vi "AlGaInPAs_prep_run_cont_dil_v13.vi"(2 "Debug Mode":bool, 3 "Elapsed Time(s)":dbl, 4 "State":enum16{"Edit", "Start", "Run", "End", "Idle"}(ring), 5 "Argument List In":string[](array[string])) -> (0 "Status Out":string, 1 "Argument List Out":string[](array[string]))   [LabVIEW 2011]
panel:
  out "Prep-In var":bool
  out "Prep-Ga var":bool
  out "Prep-Al var":bool
  out "Prep-P var":bool
  out "Prep-As var":bool
  out "prep_done":bool
  out "run started":bool
  out "first":bool=TRUE
  out "total time":dbl
  out "is OK?":bool
  out "AsH3?":bool
  out "PH3?":bool
  out "In?":bool
  out "Ga?":bool
  out "Al?":bool
  in  "Prep As":bool caption="Pre-run"
  in  "Prep P":bool caption="Pre-run"
  in  "Prep In":bool caption="Pre-run"
  in  "prep_time":dbl caption="pre-run time (s)"
  in  "Prep Al":bool caption="Pre-run"
  in  "Run As":bool caption="Run"
  in  "AsH3 Flow":dbl caption="AsH3 Flow (0-10 sccm)" format="%.2f"
  in  "P Flow":dbl caption="P Flow (0-100 sccm)" format="%.2f"
  in  "Run P":bool caption="Run"
  in  "In Flow":dbl caption="In Flow (0-100 sscm)" format="%.2f"
  in  "Run In":bool caption="Run"
  in  "Run Al":bool caption="Run"
  in  "Al Flow":dbl caption="Al Flow (0-100 sscm)" format="%.2f"
  in  "Cancel":bool
  in  "OK":bool
  out "tTotal(s) 2":dbl
  in  "Ga Tab Control":enum32{"Page 1", "Page 2", "Page 3"}(tab)
  in  "Ga Dilution":bool caption="Dilute"
  in  "Ga Flow set":dbl caption="Ga Flow (0-10 sscm)" format="%.2f"
  in  "Run Ga":bool caption="Run"
  in  "Prep Ga":bool caption="Pre-run"
  out "Ga Flow val":dbl caption="Ga Flow (0-10 sscm)" format="%.2f"
  in  "GAMFC1 set":dbl=1.0 caption="R1 (0-10 sscm)" format="%.2f"
  out "GAMFC2 val":dbl caption="R2 (0-100 sscm)" format="%.2f"
  in  "GAMFC3 set":dbl=100.0 caption="R3 (0-1000 sscm)" format="%.1f"
  out "GAMFC1 val":dbl caption="R1 (0-10 sscm)" format="%.2f"
  in  "GAMFC2 set":dbl caption="R2 (0-100 sscm)" format="%.2f"
  out "GAMFC3 val":dbl=100.0 caption="R3 (0-1000 sscm)" format="%.1f"
  in  "Ga calculated":u16(ring) items=["Ga flow", "MFC1", "MFC2", "MFC3"]
  # "Add pre-run time to run time in editor."
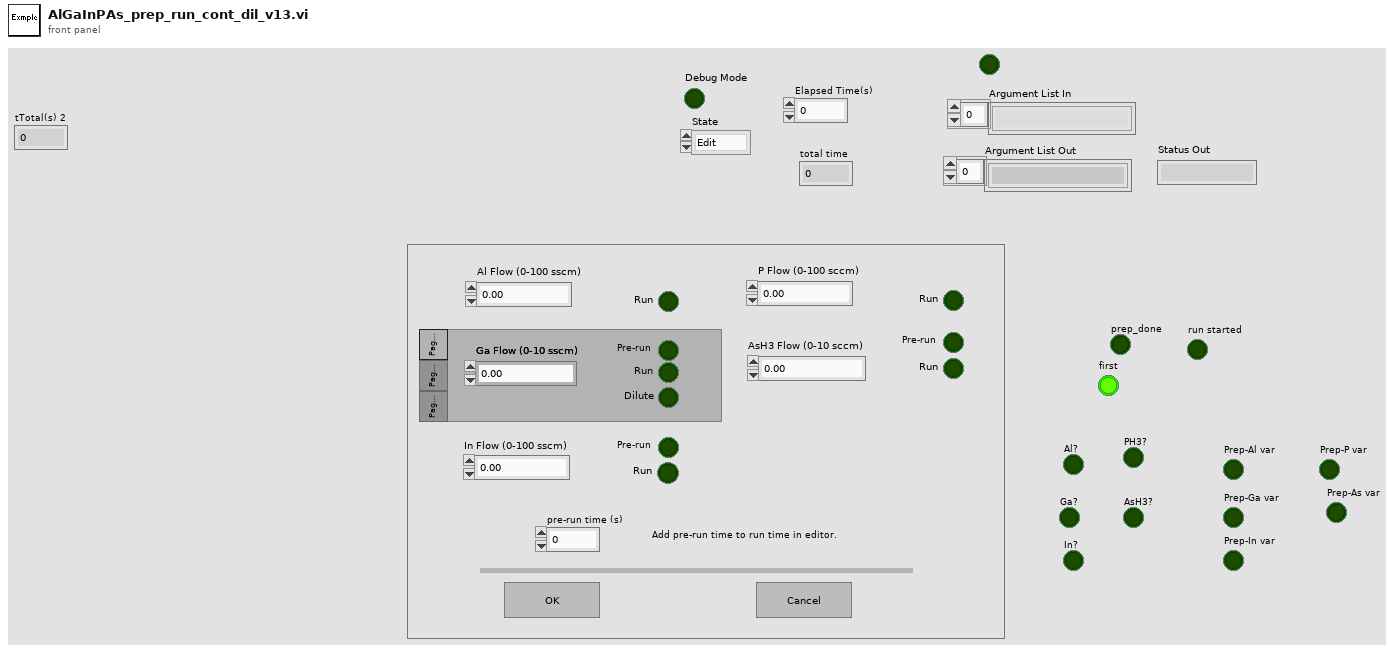
[diagram p1: front panel]
types:
  T1 = enum16{"Discrete", "Continuous", "Instantaneous", "Finite"}
  T2 = enum32{"Invalid", "Default", "Floating", "Floating/Auto-Hide", "Modal"}
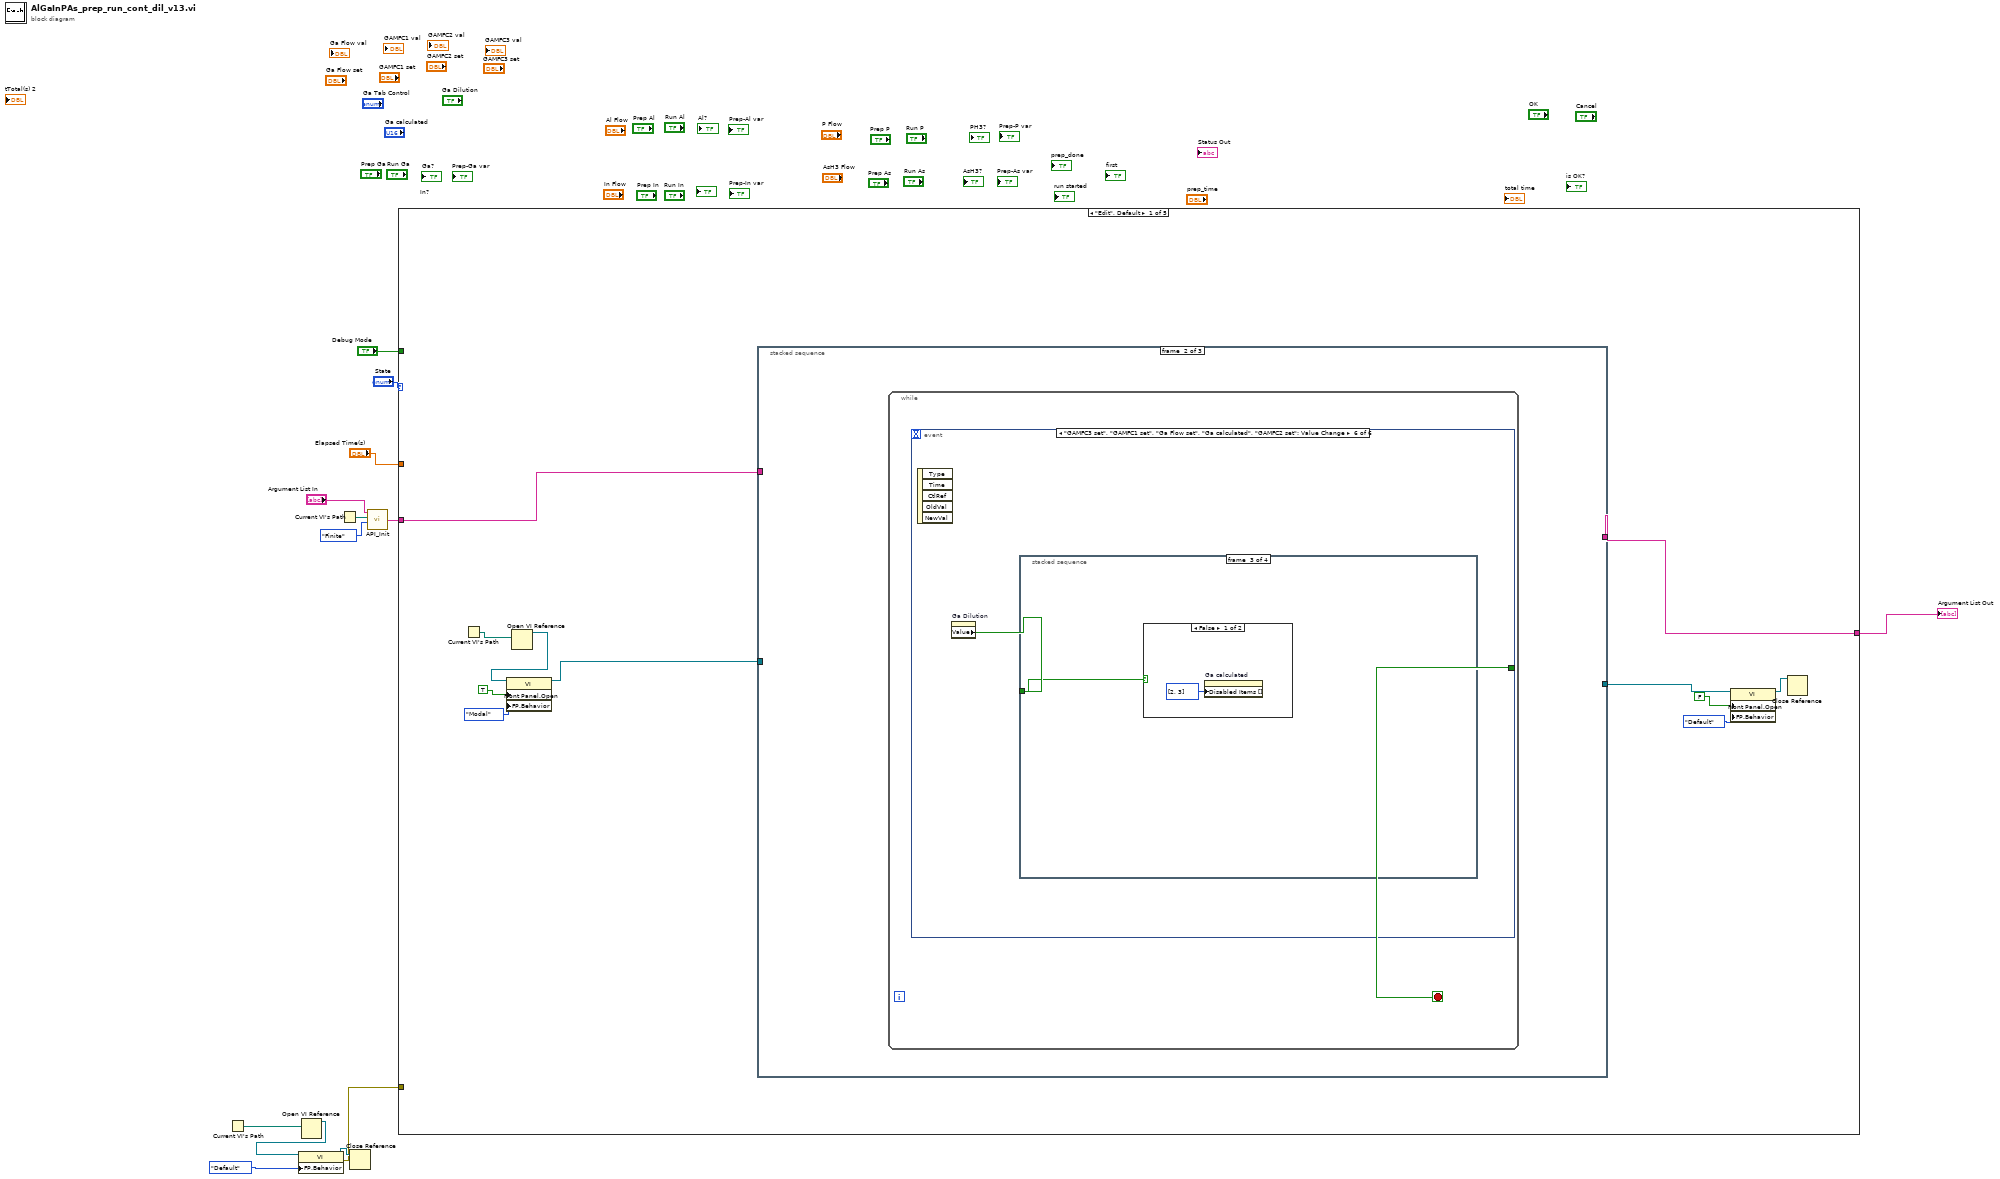
[diagram p0: block diagram]
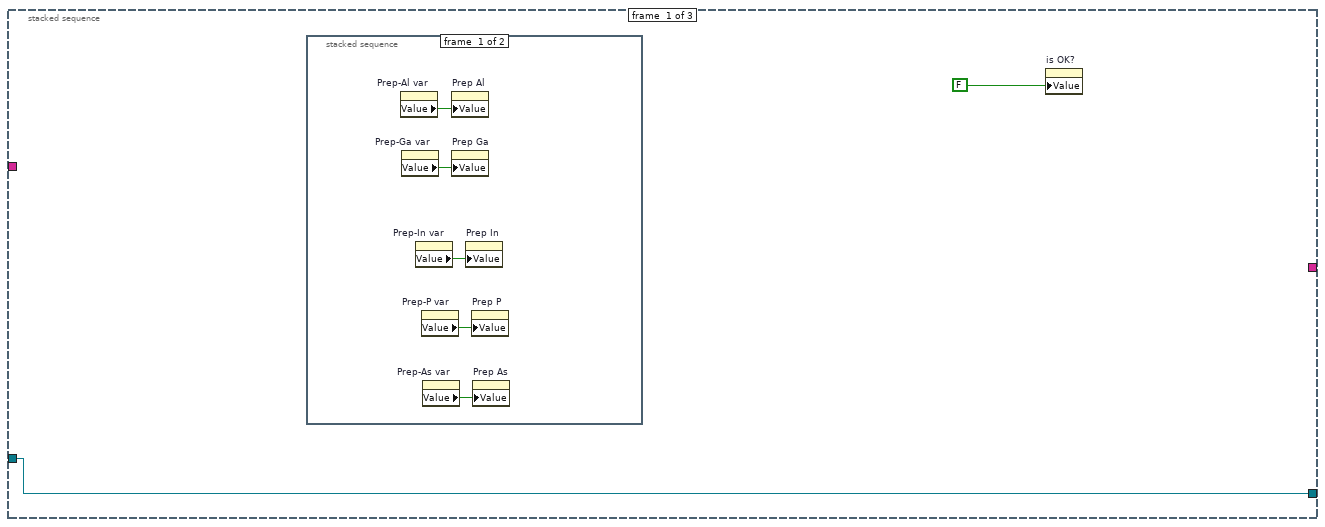
[diagram p2: hidden frame]
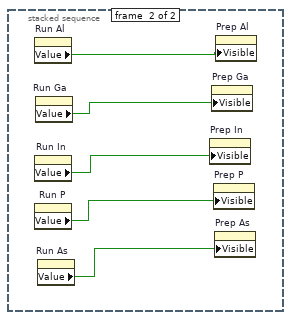
[diagram p3: hidden frame]
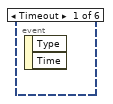
[diagram p4: hidden frame]
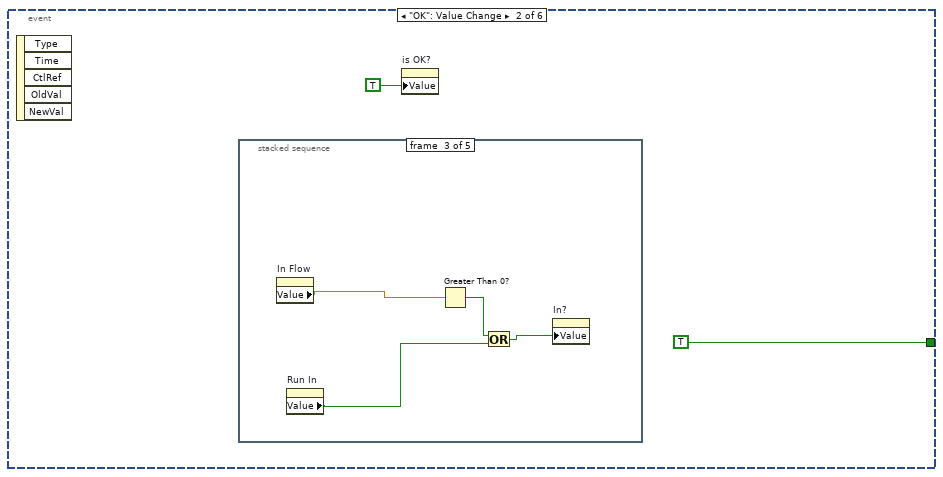
[diagram p5: hidden frame]
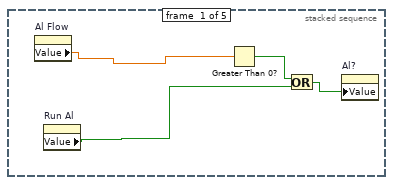
[diagram p6: hidden frame]
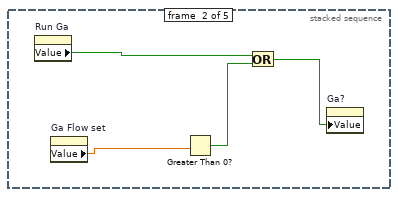
[diagram p7: hidden frame]
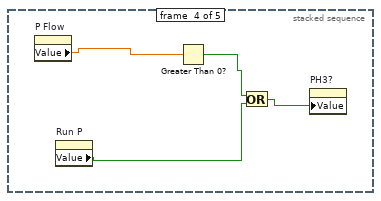
[diagram p8: hidden frame]
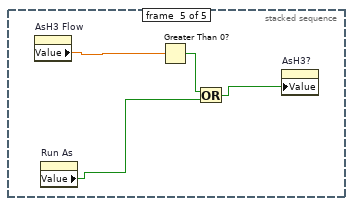
[diagram p9: hidden frame]
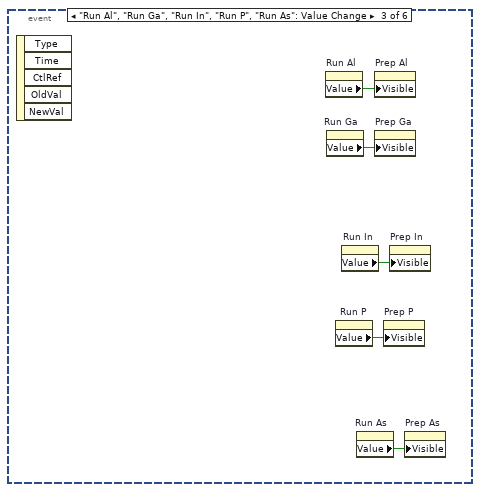
[diagram p10: hidden frame]
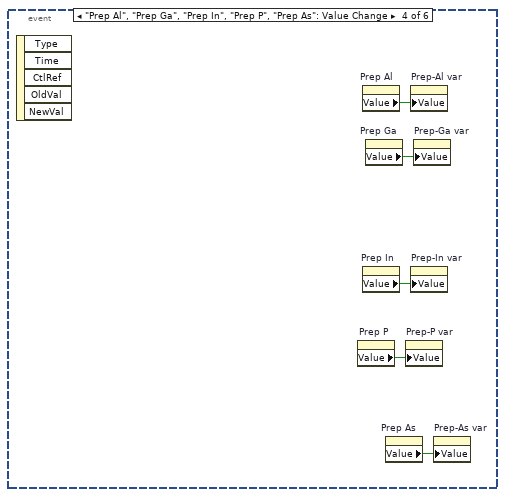
[diagram p11: hidden frame]
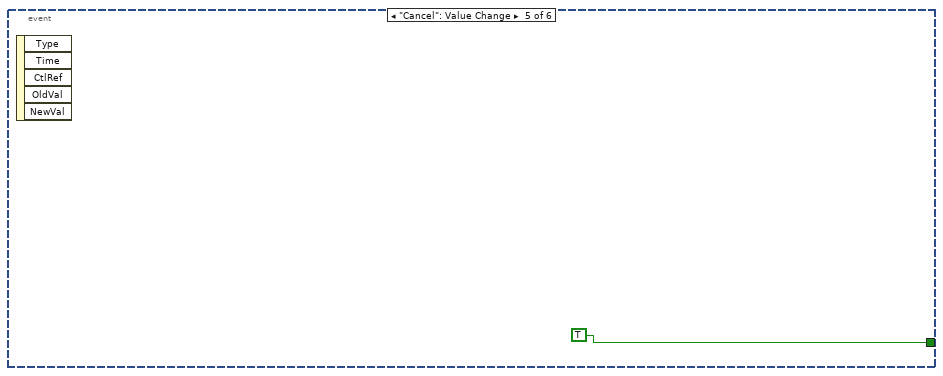
[diagram p12: hidden frame]
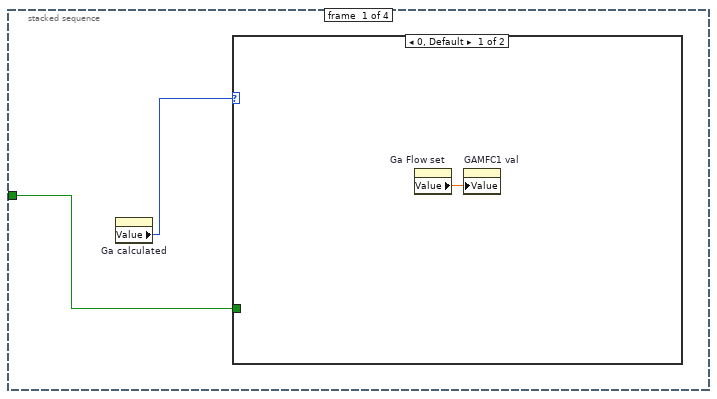
[diagram p13: hidden frame]
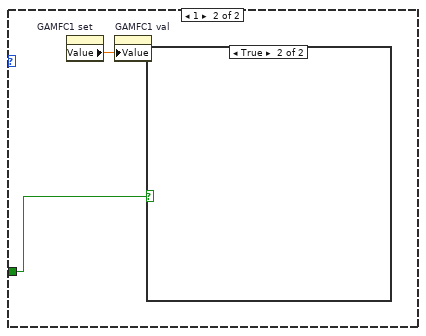
[diagram p14: hidden frame]
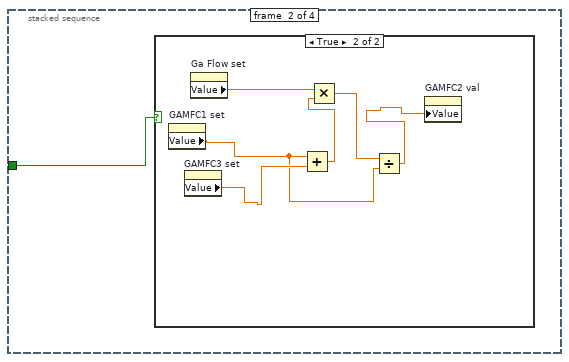
[diagram p16: hidden frame]
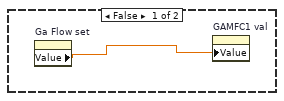
[diagram p17: hidden frame]
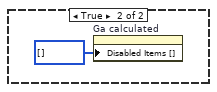
[diagram p18: hidden frame]
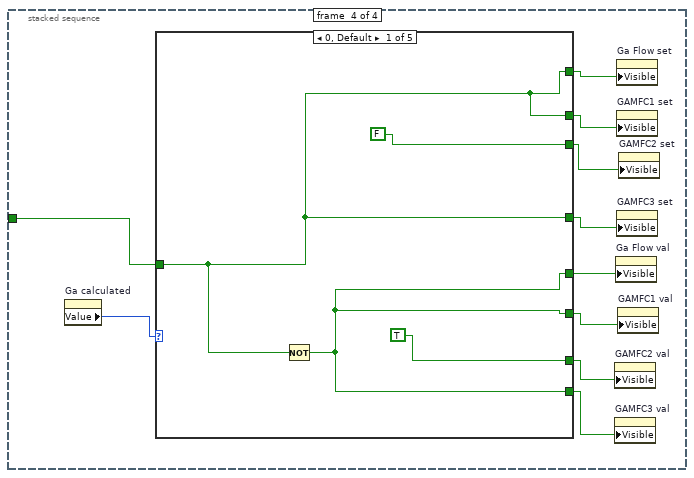
[diagram p19: hidden frame]
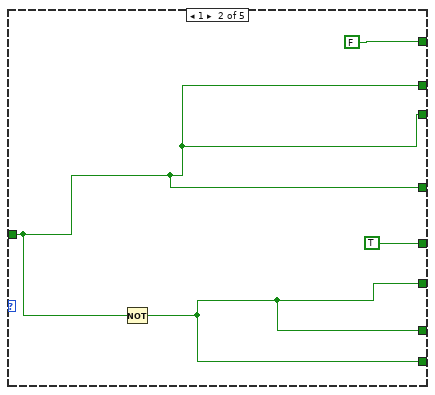
[diagram p20: hidden frame]
diagram:
  n1 = Current VI's Path() -> (path=w9:path)
  n2 = Open VI Reference(vi path=w9) -> (vi reference=w8:refnum<vi>)  [unwired: 1 in, 5 out]
  n3 = property class="VI"(reference=w8, "FP.Behavior"=T2."Default" ("Front Panel Window:Behavior")) -> (reference out=w6:refnum<vi>, error out=w5:errorcluster)  [unwired: 1 in]
  n4 = Current VI's Path() -> (path=w4:path)
  n5 = Close Reference(reference=w6) -> ()  [unwired: 1 in, 1 out]
  n6 = call "API_Init.vi"("API Mode"=T1."Finite", "VI Path"=w4, "Argument List In"="Argument List In") -> ("Argument List Out"=w1:string[])  [unwired: 1 in]
  n7 = case shown="\"Edit\", Default" "State" {
    tunnel: "Debug Mode" -> [_ w126 w183 _ _]
    tunnel: "Elapsed Time(s)" -> [_ _ w185 _ _]
    tunnel: w1 -> [w15 w128 w182 w302 w303]
    tunnel: [w14 w127 w184 w302 w303] -> w10
    tunnel: w5 -> [_ _ _ _ _]
    frame "Edit", Default {
      n8 = Current VI's Path() -> (path=w20:path)
      n9 = Open VI Reference(vi path=w20) -> (vi reference=w19:refnum<vi>)  [unwired: 1 in, 5 out]
      n10 = property class="VI"(reference=w19, "Front Panel.Open"=TRUE ("Front Panel Window:Open"), "FP.Behavior"=T2."Modal" ("Front Panel Window:Behavior")) -> (reference out=w18:refnum<vi>)  [unwired: 1 in, 1 out]
      n11 = stacked-sequence {
        tunnel: w15 -> [_ _ w121]
        tunnel: w18 -> [w26 _ _]
        tunnel: [w26 _ _] -> w22
        tunnel: [_ _ w119] -> w14
        frame #0 {
          n12 = stacked-sequence {
            frame #0 {
              n13 = property on="Prep-Al var" class="Bool (strict)"() -> ("Value"=w31:bool)  [unwired: 2 in, 2 out]
              n14 = property on="Prep-Ga var" class="Bool (strict)"() -> ("Value"=w30:bool)  [unwired: 2 in, 2 out]
              n15 = property on="Prep-In var" class="Bool (strict)"() -> ("Value"=w29:bool)  [unwired: 2 in, 2 out]
              n16 = property on="Prep-P var" class="Bool (strict)"() -> ("Value"=w28:bool)  [unwired: 2 in, 2 out]
              n17 = property on="Prep-As var" class="Bool (strict)"() -> ("Value"=w27:bool)  [unwired: 2 in, 2 out]
              n18 = property on="Prep Al" class="Bool (strict)"("Value"=w31) -> ()  [unwired: 2 in, 2 out]
              n19 = property on="Prep Ga" class="Bool (strict)"("Value"=w30) -> ()  [unwired: 2 in, 2 out]
              n20 = property on="Prep In" class="Bool (strict)"("Value"=w29) -> ()  [unwired: 2 in, 2 out]
              n21 = property on="Prep P" class="Bool (strict)"("Value"=w28) -> ()  [unwired: 2 in, 2 out]
              n22 = property on="Prep As" class="Bool (strict)"("Value"=w27) -> ()  [unwired: 2 in, 2 out]
            }
            frame #1 {
              n23 = property on="Run Al" class="Bool (strict)"() -> ("Value"=w36:bool)  [unwired: 2 in, 2 out]
              n24 = property on="Run In" class="Bool (strict)"() -> ("Value"=w34:bool)  [unwired: 2 in, 2 out]
              n25 = property on="Run P" class="Bool (strict)"() -> ("Value"=w33:bool)  [unwired: 2 in, 2 out]
              n26 = property on="Run Ga" class="Bool (strict)"() -> ("Value"=w35:bool)  [unwired: 2 in, 2 out]
              n27 = property on="Run As" class="Bool (strict)"() -> ("Value"=w32:bool)  [unwired: 2 in, 2 out]
              n28 = property on="Prep In" class="Bool (strict)"("Visible"=w34) -> ()  [unwired: 2 in, 2 out]
              n29 = property on="Prep Ga" class="Bool (strict)"("Visible"=w35) -> ()  [unwired: 2 in, 2 out]
              n30 = property on="Prep P" class="Bool (strict)"("Visible"=w33) -> ()  [unwired: 2 in, 2 out]
              n31 = property on="Prep As" class="Bool (strict)"("Visible"=w32) -> ()  [unwired: 2 in, 2 out]
              n32 = property on="Prep Al" class="Bool (strict)"("Visible"=w36) -> ()  [unwired: 2 in, 2 out]
            }
          }
          n33 = property on="is OK?" class="Bool (strict)"("Value"=FALSE ("is OK?")) -> ()  [unwired: 2 in, 2 out]
        }
        frame #1 {
          n34 = while {
            stop <- w37 stop-if-true
            n35 = event shown="[5] \"GAMFC3 set\", \"GAMFC1 set\", \"Ga Flow set\", \"Ga calculated\", \"GAMFC2 set\": Value Change" {
              selector: _ -> [_ _ _ _ _ _]
              dyn-events: _ -> [_ _ _ _ _ _]
              timeout: _ -> [_ _ _ _ _ _]
              tunnel: [_ TRUE _ _ TRUE _] -> w37
              event Timeout {
                n36 = event-data() -> ()  [unwired: 1 in, 2 out]
              }
              event "OK": Value Change {
                n37 = event-data() -> ()  [unwired: 1 in, 5 out]
                n38 = stacked-sequence {
                  frame #0 {
                    n39 = property on="Al Flow" class="DigNum (strict)"() -> ("Value"=w42:dbl)  [unwired: 2 in, 2 out]
                    n40 = property on="Run Al" class="Bool (strict)"() -> ("Value"=w41:bool)  [unwired: 2 in, 2 out]
                    n41 = Greater Than 0?(x=w42) -> (x > 0?=w43:bool)
                    n42 = Or(x=w43, y=w41) -> (x .or. y?=w40:bool)
                    n43 = property on="Al?" class="Bool (strict)"("Value"=w40) -> ()  [unwired: 2 in, 2 out]
                  }
                  frame #1 {
                    n44 = property on="Run Ga" class="Bool (strict)"() -> ("Value"=w45:bool)  [unwired: 2 in, 2 out]
                    n45 = property on="Ga Flow set" class="DigNum (strict)"() -> ("Value"=w46:dbl)  [unwired: 2 in, 2 out]
                    n46 = Greater Than 0?(x=w46) -> (x > 0?=w47:bool)
                    n47 = Or(x=w45, y=w47) -> (x .or. y?=w44:bool)
                    n48 = property on="Ga?" class="Bool (strict)"("Value"=w44) -> ()  [unwired: 2 in, 2 out]
                  }
                  frame #2 {
                    n49 = property on="In Flow" class="DigNum (strict)"() -> ("Value"=w49:dbl)  [unwired: 2 in, 2 out]
                    n50 = property on="Run In" class="Bool (strict)"() -> ("Value"=w50:bool)  [unwired: 2 in, 2 out]
                    n51 = Greater Than 0?(x=w49) -> (x > 0?=w51:bool)
                    n52 = Or(x=w51, y=w50) -> (x .or. y?=w48:bool)
                    n53 = property on="In?" class="Bool (strict)"("Value"=w48) -> ()  [unwired: 2 in, 2 out]
                  }
                  frame #3 {
                    n54 = property on="P Flow" class="DigNum (strict)"() -> ("Value"=w54:dbl)  [unwired: 2 in, 2 out]
                    n55 = property on="Run P" class="Bool (strict)"() -> ("Value"=w53:bool)  [unwired: 2 in, 2 out]
                    n56 = Greater Than 0?(x=w54) -> (x > 0?=w55:bool)
                    n57 = Or(x=w55, y=w53) -> (x .or. y?=w52:bool)
                    n58 = property on="PH3?" class="Bool (strict)"("Value"=w52) -> ()  [unwired: 2 in, 2 out]
                  }
                  frame #4 {
                    n59 = property on="AsH3 Flow" class="DigNum (strict)"() -> ("Value"=w58:dbl)  [unwired: 2 in, 2 out]
                    n60 = property on="Run As" class="Bool (strict)"() -> ("Value"=w57:bool)  [unwired: 2 in, 2 out]
                    n61 = Greater Than 0?(x=w58) -> (x > 0?=w59:bool)
                    n62 = Or(x=w59, y=w57) -> (x .or. y?=w56:bool)
                    n63 = property on="AsH3?" class="Bool (strict)"("Value"=w56) -> ()  [unwired: 2 in, 2 out]
                  }
                }
                n64 = property on="is OK?" class="Bool (strict)"("Value"=TRUE ("is OK?")) -> ()  [unwired: 2 in, 2 out]
              }
              event "Run Al", "Run Ga", "Run In", "Run P", "Run As": Value Change {
                n65 = event-data() -> ()  [unwired: 1 in, 5 out]
                n66 = property on="Run Al" class="Bool (strict)"() -> ("Value"=w64:bool)  [unwired: 2 in, 2 out]
                n67 = property on="Run Ga" class="Bool (strict)"() -> ("Value"=w63:bool)  [unwired: 2 in, 2 out]
                n68 = property on="Run P" class="Bool (strict)"() -> ("Value"=w60:bool)  [unwired: 2 in, 2 out]
                n69 = property on="Run In" class="Bool (strict)"() -> ("Value"=w62:bool)  [unwired: 2 in, 2 out]
                n70 = property on="Run As" class="Bool (strict)"() -> ("Value"=w61:bool)  [unwired: 2 in, 2 out]
                n71 = property on="Prep Al" class="Bool (strict)"("Visible"=w64) -> ()  [unwired: 2 in, 2 out]
                n72 = property on="Prep Ga" class="Bool (strict)"("Visible"=w63) -> ()  [unwired: 2 in, 2 out]
                n73 = property on="Prep P" class="Bool (strict)"("Visible"=w60) -> ()  [unwired: 2 in, 2 out]
                n74 = property on="Prep In" class="Bool (strict)"("Visible"=w62) -> ()  [unwired: 2 in, 2 out]
                n75 = property on="Prep As" class="Bool (strict)"("Visible"=w61) -> ()  [unwired: 2 in, 2 out]
              }
              event "Prep Al", "Prep Ga", "Prep In", "Prep P", "Prep As": Value Change {
                n76 = event-data() -> ()  [unwired: 1 in, 5 out]
                n77 = property on="Prep P" class="Bool (strict)"() -> ("Value"=w66:bool)  [unwired: 2 in, 2 out]
                n78 = property on="Prep Al" class="Bool (strict)"() -> ("Value"=w69:bool)  [unwired: 2 in, 2 out]
                n79 = property on="Prep In" class="Bool (strict)"() -> ("Value"=w67:bool)  [unwired: 2 in, 2 out]
                n80 = property on="Prep Ga" class="Bool (strict)"() -> ("Value"=w68:bool)  [unwired: 2 in, 2 out]
                n81 = property on="Prep As" class="Bool (strict)"() -> ("Value"=w65:bool)  [unwired: 2 in, 2 out]
                n82 = property on="Prep-P var" class="Bool (strict)"("Value"=w66) -> ()  [unwired: 2 in, 2 out]
                n83 = property on="Prep-Al var" class="Bool (strict)"("Value"=w69) -> ()  [unwired: 2 in, 2 out]
                n84 = property on="Prep-In var" class="Bool (strict)"("Value"=w67) -> ()  [unwired: 2 in, 2 out]
                n85 = property on="Prep-Ga var" class="Bool (strict)"("Value"=w68) -> ()  [unwired: 2 in, 2 out]
                n86 = property on="Prep-As var" class="Bool (strict)"("Value"=w65) -> ()  [unwired: 2 in, 2 out]
              }
              event "Cancel": Value Change {
                n87 = event-data() -> ()  [unwired: 1 in, 5 out]
              }
              event "GAMFC3 set", "GAMFC1 set", "Ga Flow set", "Ga calculated", "GAMFC2 set": Value Change {
                n88 = event-data() -> ()  [unwired: 1 in, 5 out]
                n89 = property on="Ga Dilution" class="Bool (strict)"() -> ("Value"=w71:bool)  [unwired: 2 in, 2 out]
                n90 = stacked-sequence {
                  tunnel: w71 -> [w72 w77 w85 w96]
                  frame #0 {
                    n91 = property on="Ga calculated" class="Ring (strict)"() -> ("Value"=w73:u16)  [unwired: 2 in, 2 out]
                    n92 = case shown="0, Default" w73 {
                      tunnel: w72 -> [_ w75]
                      frame 0, Default {
                        n93 = property on="Ga Flow set" class="DigNum (strict)"() -> ("Value"=w74:dbl)  [unwired: 2 in, 2 out]
                        n94 = property on="GAMFC1 val" class="DigNum (strict)"("Value"=w74) -> ()  [unwired: 2 in, 2 out]
                      }
                      frame 1 {
                        n95 = property on="GAMFC1 set" class="DigNum (strict)"() -> ("Value"=w76:dbl)  [unwired: 2 in, 2 out]
                        n96 = property on="GAMFC1 val" class="DigNum (strict)"("Value"=w76) -> ()  [unwired: 2 in, 2 out]
                        n97 = case shown="True" w75 {
                          frame False {
                          }
                          frame True {
                          }
                        }
                      }
                    }
                  }
                  frame #1 {
                    n98 = case shown="True" w77 {
                      frame False {
                        n99 = property on="Ga Flow set" class="DigNum (strict)"() -> ("Value"=w78:dbl)  [unwired: 2 in, 2 out]
                        n100 = property on="GAMFC1 val" class="DigNum (strict)"("Value"=w78) -> ()  [unwired: 2 in, 2 out]
                      }
                      frame True {
                        n101 = property on="GAMFC1 set" class="DigNum (strict)"() -> ("Value"=w79:dbl)  [unwired: 2 in, 2 out]
                        n102 = property on="GAMFC3 set" class="DigNum (strict)"() -> ("Value"=w81:dbl)  [unwired: 2 in, 2 out]
                        n103 = property on="Ga Flow set" class="DigNum (strict)"() -> ("Value"=w82:dbl)  [unwired: 2 in, 2 out]
                        n104 = Add(x=w79, y=w81) -> (x+y=w84:dbl)
                        n105 = Multiply(x=w82, y=w84) -> (x*y=w80:dbl)
                        n106 = Divide(x=w80, y=w79) -> (x/y=w83:dbl)
                        n107 = property on="GAMFC2 val" class="DigNum (strict)"("Value"=w83) -> ()  [unwired: 2 in, 2 out]
                      }
                    }
                  }
                  frame #2 {
                    n108 = case shown="False" w85 {
                      frame False {
                        n109 = property on="Ga calculated" class="Ring (strict)"("Disabled Items []"=i32[] [2, 3]) -> ()  [unwired: 2 in, 2 out]
                      }
                      frame True {
                        n110 = property on="Ga calculated" class="Ring (strict)"("Disabled Items []"=i32[] []) -> ()  [unwired: 2 in, 2 out]
                      }
                    }
                  }
                  frame #3 {
                    n111 = property on="Ga calculated" class="Ring (strict)"() -> ("Value"=w97:u16)  [unwired: 2 in, 2 out]
                    n112 = case shown="0, Default" w97 {
                      tunnel: w96 -> [w99 w104 w107 w111 w115]
                      tunnel: [w99 FALSE ("Visible") w107 w111 w115] -> w95
                      tunnel: [w99 w104 FALSE ("Visible") w111 w115] -> w93
                      tunnel: [FALSE ("Visible") w104 w107 FALSE ("Visible") w115] -> w94
                      tunnel: [w99 w104 w107 w111 FALSE ("Visible")] -> w92
                      tunnel: [w98 w103 TRUE ("Visible") w110 w114] -> w90
                      tunnel: [TRUE ("Visible") w103 w106 TRUE ("Visible") w114] -> w89
                      tunnel: [w98 w103 w106 w110 TRUE ("Visible")] -> w88
                      tunnel: [w98 TRUE ("Visible") w106 w110 w114] -> w91
                      frame 0, Default {
                        n113 = Not(x=w99) -> (.not. x?=w98:bool)
                      }
                      frame 1 {
                        n114 = Not(x=w104) -> (.not. x?=w103:bool)
                      }
                      frame 2 {
                        n115 = Not(x=w107) -> (.not. x?=w106:bool)
                      }
                      frame 3 {
                        n116 = Not(x=w111) -> (.not. x?=w110:bool)
                      }
                      frame 4 {
                        n117 = Not(x=w115) -> (.not. x?=w114:bool)
                      }
                    }
                    n118 = property on="GAMFC2 val" class="DigNum (strict)"("Visible"=w89) -> ()  [unwired: 2 in, 2 out]
                    n119 = property on="GAMFC3 val" class="DigNum (strict)"("Visible"=w88) -> ()  [unwired: 2 in, 2 out]
                    n120 = property on="Ga Flow val" class="DigNum (strict)"("Visible"=w91) -> ()  [unwired: 2 in, 2 out]
                    n121 = property on="Ga Flow set" class="DigNum (strict)"("Visible"=w95) -> ()  [unwired: 2 in, 2 out]
                    n122 = property on="GAMFC1 set" class="DigNum (strict)"("Visible"=w93) -> ()  [unwired: 2 in, 2 out]
                    n123 = property on="GAMFC3 set" class="DigNum (strict)"("Visible"=w92) -> ()  [unwired: 2 in, 2 out]
                    n124 = property on="GAMFC1 val" class="DigNum (strict)"("Visible"=w90) -> ()  [unwired: 2 in, 2 out]
                    n125 = property on="GAMFC2 set" class="DigNum (strict)"("Visible"=w94) -> ()  [unwired: 2 in, 2 out]
                  }
                }
              }
            }
          }
        }
        frame #2 {
          n126 = property on="is OK?" class="Bool (strict)"() -> ("Value"=w118:bool)  [unwired: 2 in, 2 out]
          n127 = case shown="True" w118 {
            tunnel: w121 -> [w124 w125]
            tunnel: [w124 w125] -> w120
            frame False {
            }
            frame True {
            }
          }
          n128 = Not(x=w118) -> (.not. x?=w123:bool)
          n129 = Current VI's Path() -> (path=w122:path)
          n130 = call "API_Edit.vi"("Cancel"=w123, "OK"=w118, "VI Path"=w122, "Argument List In"=w120) -> ("Argument List Out"=w119:string[])
        }
      }
      n131 = property class="VI"(reference=w22, "Front Panel.Open"=FALSE ("Front Panel Window:Open"), "FP.Behavior"=T2."Default" ("Front Panel Window:Behavior")) -> (reference out=w23:refnum<vi>)  [unwired: 1 in, 1 out]
      n132 = Close Reference(reference=w23) -> ()  [unwired: 1 in, 1 out]
    }
    frame "Start" {
      n133 = call "Set_Argument.vi"("Enable"=FALSE, "Argument"="run_started", "Argument List In"=w128) -> ("Argument List Out"=w127:string[])
      n134 = stacked-sequence {
        tunnel: w126 -> [w131 w140 w155 w164 w173]
        frame #0 {
          n135 = case shown="False" w131 {
            frame False {
              n136 = property on="Al?" class="Bool (strict)"() -> ("Value"=w132:bool)  [unwired: 2 in, 2 out]
              n137 = case shown="True" w132 {
                frame False {
                  w133 = FALSE ("Al Active")
                  n138 = call "set_Al.vi"("Aluminum Flow"=0.0, "Al Remote"=w133, "Al Run"=w133, "Al Bubbler"=w133, "Al Active"=w133) -> ()  [unwired: 5 out]
                }
                frame True {
                  w139 = TRUE ("Al Active")
                  n139 = property on="Prep Al" class="Bool (strict)"() -> ("Value"=w137:bool)  [unwired: 2 in, 2 out]
                  n140 = property on="Run Al" class="Bool (strict)"() -> ("Value"=w136:bool)  [unwired: 2 in, 2 out]
                  n141 = property on="Al Flow" class="DigNum (strict)"() -> ("Value"=w138:dbl)  [unwired: 2 in, 2 out]
                  n142 = And(x=w137, y=w136) -> (x .and. y?=w135:bool)
                  n143 = call "set_Al.vi"("Aluminum Flow"=w138, "Al Run"=w135, "Al Bubbler"=w139, "Al Active"=w139) -> ()  [unwired: 1 in, 5 out]
                }
              }
            }
            frame True {
            }
          }
        }
        frame #1 {
          n144 = case shown="False" w140 {
            frame False {
              n145 = property on="Ga?" class="Bool (strict)"() -> ("Value"=w141:bool)  [unwired: 2 in, 2 out]
              n146 = case shown="True" w141 {
                frame False {
                  w143 = FALSE ("Ga Active")
                  w142 = 0.0 ("Ga Flow 1")
                  n147 = call "set_Ga.vi"("Ga Active"=w143, "Ga Flow 3"=w142, "Ga Flow 2"=w142, "Ga Flow 1"=w142, "Ga Bubbler"=w143, "Ga H2 Dilute"=w143, "Ga Run"=w143, "Ga Remote"=w143) -> ()  [unwired: 8 out]
                }
                frame True {
                  w146 = TRUE ("Ga Active")
                  n148 = property on="Ga Dilution" class="Bool (strict)"() -> ("Value"=w145:bool)  [unwired: 2 in, 2 out]
                  n149 = property on="GAMFC2 val" class="DigNum (strict)"() -> ("Value"=w148:dbl)  [unwired: 2 in, 2 out]
                  n150 = property on="GAMFC3 set" class="DigNum (strict)"() -> ("Value"=w147:dbl)  [unwired: 2 in, 2 out]
                  n151 = property on="Prep-Ga var" class="Bool (strict)"() -> ("Value"=w149:bool)  [unwired: 2 in, 2 out]
                  n152 = property on="Run Ga" class="Bool (strict)"() -> ("Value"=w150:bool)  [unwired: 2 in, 2 out]
                  n153 = case shown="True" w145 {
                    tunnel: [w153 w154] -> w144
                    frame False {
                      n154 = property on="GAMFC1 val" class="DigNum (strict)"() -> ("Value"=w153:dbl)  [unwired: 2 in, 2 out]
                    }
                    frame True {
                      n155 = property on="GAMFC1 set" class="DigNum (strict)"() -> ("Value"=w154:dbl)  [unwired: 2 in, 2 out]
                    }
                  }
                  n156 = And(x=w149, y=w150) -> (x .and. y?=w152:bool)
                  n157 = property on="Ga Dilution" class="Bool (strict)"() -> ("Value"=w151:bool)  [unwired: 2 in, 2 out]
                  n158 = call "set_Ga.vi"("Ga Active"=w146, "Ga Flow 3"=w147, "Ga Flow 2"=w148, "Ga Flow 1"=w144, "Ga Bubbler"=w146, "Ga H2 Dilute"=w151, "Ga Run"=w152, "Ga Remote"=w146) -> ()  [unwired: 8 in]
                }
              }
            }
            frame True {
            }
          }
        }
        frame #2 {
          n159 = case shown="False" w155 {
            frame False {
              n160 = property on="In?" class="Bool (strict)"() -> ("Value"=w156:bool)  [unwired: 2 in, 2 out]
              n161 = case shown="True" w156 {
                frame False {
                  w158 = FALSE ("In Remote")
                  n162 = call "set_In.vi"("Indium Flow"=0.0, "In Remote"=w158, "In Run"=w158, "In Bubbler"=w158, "In Active"=w158) -> ()  [unwired: 5 out]
                }
                frame True {
                  w163 = TRUE ("In Run")
                  n163 = property on="Run In" class="Bool (strict)"() -> ("Value"=w160:bool)  [unwired: 2 in, 2 out]
                  n164 = property on="Prep In" class="Bool (strict)"() -> ("Value"=w161:bool)  [unwired: 2 in, 2 out]
                  n165 = And(x=w161, y=w160) -> (x .and. y?=w159:bool)
                  n166 = property on="In Flow" class="DigNum (strict)"() -> ("Value"=w162:dbl)  [unwired: 2 in, 2 out]
                  n167 = call "set_In.vi"("Indium Flow"=w162, "In Run"=w159, "In Bubbler"=w163, "In Active"=w163) -> ()  [unwired: 1 in, 5 out]
                }
              }
            }
            frame True {
            }
          }
        }
        frame #3 {
          n168 = case shown="False" w164 {
            frame False {
              n169 = property on="PH3?" class="Bool (strict)"() -> ("Value"=w165:bool)  [unwired: 2 in, 2 out]
              n170 = case shown="True" w165 {
                frame False {
                  w166 = FALSE ("P_Gas Active")
                  n171 = call "set_P_gas.vi"("P_Gas Active"=w166, "P_Gas Flow"=0.0, "P_Gas In"=w166, "P_Gas H2 In"=w166, "P_Gas Run"=w166, "P_Gas Remote"=w166) -> ()  [unwired: 10 out]
                }
                frame True {
                  w172 = TRUE ("P_Gas Active")
                  n172 = property on="P Flow" class="DigNum (strict)"() -> ("Value"=w171:dbl)  [unwired: 2 in, 2 out]
                  n173 = property on="Prep P" class="Bool (strict)"() -> ("Value"=w170:bool)  [unwired: 2 in, 2 out]
                  n174 = property on="Run P" class="Bool (strict)"() -> ("Value"=w169:bool)  [unwired: 2 in, 2 out]
                  n175 = And(x=w170, y=w169) -> (x .and. y?=w168:bool)
                  n176 = call "set_P_gas.vi"("P_Gas Active"=w172, "P_Gas Flow"=w171, "P_Gas In"=w172, "P_Gas Run"=w168) -> ()  [unwired: 2 in, 10 out]
                }
              }
            }
            frame True {
            }
          }
        }
        frame #4 {
          n177 = case shown="False" w173 {
            frame False {
              n178 = property on="AsH3?" class="Bool (strict)"() -> ("Value"=w174:bool)  [unwired: 2 in, 2 out]
              n179 = case shown="True" w174 {
                frame False {
                  w175 = FALSE ("As_Gas Active")
                  n180 = call "set_As_gas.vi"("As_Gas Active"=w175, "As_Gas Flow"=0.0, "As_Gas In"=w175, "As_Gas H2"=w175, "As_Gas Run"=w175, "As_Gas Remote"=w175) -> ()  [unwired: 10 in]
                }
                frame True {
                  w181 = TRUE ("As_Gas Active")
                  n181 = property on="Prep As" class="Bool (strict)"() -> ("Value"=w178:bool)  [unwired: 2 in, 2 out]
                  n182 = property on="Run As" class="Bool (strict)"() -> ("Value"=w179:bool)  [unwired: 2 in, 2 out]
                  n183 = property on="AsH3 Flow" class="DigNum (strict)"() -> ("Value"=w180:dbl)  [unwired: 2 in, 2 out]
                  n184 = And(x=w178, y=w179) -> (x .and. y?=w177:bool)
                  n185 = call "set_As_gas.vi"("As_Gas Active"=w181, "As_Gas Flow"=w180, "As_Gas In"=w181, "As_Gas Run"=w177) -> ()  [unwired: 12 in]
                }
              }
            }
            frame True {
            }
          }
        }
      }
    }
    frame "Run" {
      n186 = stacked-sequence {
        tunnel: w185 -> [_ w190 _ _]
        tunnel: w182 -> [w187 _ _ w244]
        tunnel: [_ _ _ w243] -> w184
        tunnel: w183 -> [_ _ _ w245]
        frame #0 {
          n187 = call "Get_Argument.vi"("Argument"="run_started", "Argument List"=w187) -> ("Enabled"=w186:bool)
          n188 = local write "run started"(w186) -> ()
        }
        frame #1 {
          n189 = property on="prep_time" class="DigNum (strict)"() -> ("Value"=w191:dbl)  [unwired: 2 in, 2 out]
          n190 = Greater Or Equal?(x=w190, y=w191) -> (x >= y?=w189:bool)
          n191 = local write "prep_done"(w189) -> ()
        }
        frame #2 {
          n192 = local read "run started"() -> (w193:bool)
          n193 = Not(x=w193) -> (.not. x?=w192:bool)
          n194 = stacked-sequence {
            tunnel: w192 -> [w195 w199 w208 w217 w226 w235]
            frame #0 {
              n195 = case shown="True" w195 {
                tunnel: ["run: " "pre-run: "] -> w194
                frame False {
                }
                frame True {
                }
              }
              n196 = property on="Status Out" class="Str"("Value"=w194) -> ()  [unwired: 2 in, 2 out]
            }
            frame #1 {
              n197 = property on="Status Out" class="Str"() -> ("Value"=w205:string)  [unwired: 2 in, 2 out]
              n198 = property on="Al?" class="Bool (strict)"() -> ("Value"=w206:bool)  [unwired: 2 in, 2 out]
              n199 = property on="Run Al" class="Bool (strict)"() -> ("Value"=w198:bool)  [unwired: 2 in, 2 out]
              n200 = property on="Prep Al" class="Bool (strict)"() -> ("Value"=w200:bool)  [unwired: 2 in, 2 out]
              n201 = call "flow_strings.vi"("string in"=w205, "is first in?"=TRUE, "use source?"=w206, "name"="Al", "run source?"=w198, "prep source?"=w200, "is prep?"=w199) -> ("string out"=w204:string, "is first out?"=w203:bool)
              n202 = property on="Status Out" class="Str"("Value"=w204) -> ()  [unwired: 2 in, 2 out]
              n203 = property on="first" class="Bool (strict)"("Value"=w203) -> ()  [unwired: 2 in, 2 out]
            }
            frame #2 {
              n204 = property on="first" class="Bool (strict)"() -> ("Value"=w211:bool)  [unwired: 2 in, 2 out]
              n205 = property on="Status Out" class="Str"() -> ("Value"=w214:string)  [unwired: 2 in, 2 out]
              n206 = property on="Ga?" class="Bool (strict)"() -> ("Value"=w212:bool)  [unwired: 2 in, 2 out]
              n207 = property on="Run Ga" class="Bool (strict)"() -> ("Value"=w207:bool)  [unwired: 2 in, 2 out]
              n208 = property on="Prep Ga" class="Bool (strict)"() -> ("Value"=w209:bool)  [unwired: 2 in, 2 out]
              n209 = call "flow_strings.vi"("string in"=w214, "is first in?"=w211, "use source?"=w212, "name"="Ga", "run source?"=w207, "prep source?"=w209, "is prep?"=w208) -> ("string out"=w215:string, "is first out?"=w210:bool)
              n210 = property on="Status Out" class="Str"("Value"=w215) -> ()  [unwired: 2 in, 2 out]
              n211 = property on="first" class="Bool (strict)"("Value"=w210) -> ()  [unwired: 2 in, 2 out]
            }
            frame #3 {
              n212 = property on="first" class="Bool (strict)"() -> ("Value"=w221:bool)  [unwired: 2 in, 2 out]
              n213 = property on="Status Out" class="Str"() -> ("Value"=w223:string)  [unwired: 2 in, 2 out]
              n214 = property on="In?" class="Bool (strict)"() -> ("Value"=w224:bool)  [unwired: 2 in, 2 out]
              n215 = property on="Run In" class="Bool (strict)"() -> ("Value"=w216:bool)  [unwired: 2 in, 2 out]
              n216 = property on="Prep In" class="Bool (strict)"() -> ("Value"=w218:bool)  [unwired: 2 in, 2 out]
              n217 = call "flow_strings.vi"("string in"=w223, "is first in?"=w221, "use source?"=w224, "name"="In", "run source?"=w216, "prep source?"=w218, "is prep?"=w217) -> ("string out"=w220:string, "is first out?"=w219:bool)
              n218 = property on="Status Out" class="Str"("Value"=w220) -> ()  [unwired: 2 in, 2 out]
              n219 = property on="first" class="Bool (strict)"("Value"=w219) -> ()  [unwired: 2 in, 2 out]
            }
            frame #4 {
              n220 = property on="first" class="Bool (strict)"() -> ("Value"=w229:bool)  [unwired: 2 in, 2 out]
              n221 = property on="Status Out" class="Str"() -> ("Value"=w231:string)  [unwired: 2 in, 2 out]
              n222 = property on="PH3?" class="Bool (strict)"() -> ("Value"=w232:bool)  [unwired: 2 in, 2 out]
              n223 = property on="Run P" class="Bool (strict)"() -> ("Value"=w225:bool)  [unwired: 2 in, 2 out]
              n224 = property on="Prep P" class="Bool (strict)"() -> ("Value"=w227:bool)  [unwired: 2 in, 2 out]
              n225 = call "flow_strings.vi"("string in"=w231, "is first in?"=w229, "use source?"=w232, "name"="P", "run source?"=w225, "prep source?"=w227, "is prep?"=w226) -> ("string out"=w230:string, "is first out?"=w228:bool)
              n226 = property on="Status Out" class="Str"("Value"=w230) -> ()  [unwired: 2 in, 2 out]
              n227 = property on="first" class="Bool (strict)"("Value"=w228) -> ()  [unwired: 2 in, 2 out]
            }
            frame #5 {
              n228 = property on="first" class="Bool (strict)"() -> ("Value"=w238:bool)  [unwired: 2 in, 2 out]
              n229 = property on="Status Out" class="Str"() -> ("Value"=w240:string)  [unwired: 2 in, 2 out]
              n230 = property on="AsH3?" class="Bool (strict)"() -> ("Value"=w241:bool)  [unwired: 2 in, 2 out]
              n231 = property on="Run As" class="Bool (strict)"() -> ("Value"=w234:bool)  [unwired: 2 in, 2 out]
              n232 = property on="Prep As" class="Bool (strict)"() -> ("Value"=w236:bool)  [unwired: 2 in, 2 out]
              n233 = call "flow_strings.vi"("string in"=w240, "is first in?"=w238, "use source?"=w241, "name"="As", "run source?"=w234, "prep source?"=w236, "is prep?"=w235) -> ("string out"=w237:string, "is first out?"=w239:bool)
              n234 = property on="Status Out" class="Str"("Value"=w237) -> ()  [unwired: 2 in, 2 out]
              n235 = property on="first" class="Bool (strict)"("Value"=w239) -> ()  [unwired: 2 in, 2 out]
            }
          }
        }
        frame #3 {
          n236 = local read "run started"() -> (w248:bool)
          n237 = local read "prep_done"() -> (w246:bool)
          n238 = Not(x=w248) -> (.not. x?=w249:bool)
          n239 = And(x=w246, y=w249) -> (x .and. y?=w247:bool)
          n240 = stacked-sequence {
            tunnel: w247 -> [w253]
            tunnel: w245 -> [w252]
            tunnel: w244 -> [w251]
            tunnel: [w250] -> w243
            frame #0 {
              n241 = case shown="True" w253 {
                tunnel: w252 -> [_ w257]
                tunnel: w251 -> [w254 w256]
                tunnel: [w254 w255] -> w250
                frame False {
                }
                frame True {
                  n242 = stacked-sequence {
                    tunnel: w257 -> [w258 w265 w277 w284 w291 _]
                    tunnel: w256 -> [_ _ _ _ _ w299]
                    tunnel: [_ _ _ _ _ w298] -> w255
                    frame #0 {
                      n243 = case shown="False" w258 {
                        frame False {
                          n244 = property on="Al?" class="Bool (strict)"() -> ("Value"=w259:bool)  [unwired: 2 in, 2 out]
                          n245 = case shown="True" w259 {
                            frame False {
                              w260 = FALSE ("Al Active")
                              n246 = call "set_Al.vi"("Aluminum Flow"=0.0, "Al Remote"=w260, "Al Run"=w260, "Al Bubbler"=w260, "Al Active"=w260) -> ()  [unwired: 5 out]
                            }
                            frame True {
                              w264 = TRUE ("Al Active")
                              n247 = property on="Al Flow" class="DigNum (strict)"() -> ("Value"=w263:dbl)  [unwired: 2 in, 2 out]
                              n248 = property on="Run Al" class="Bool (strict)"() -> ("Value"=w262:bool)  [unwired: 2 in, 2 out]
                              n249 = call "set_Al.vi"("Aluminum Flow"=w263, "Al Run"=w262, "Al Bubbler"=w264, "Al Active"=w264) -> ()  [unwired: 1 in, 5 out]
                            }
                          }
                        }
                        frame True {
                        }
                      }
                    }
                    frame #1 {
                      n250 = case shown="False" w265 {
                        frame False {
                          n251 = property on="Ga?" class="Bool (strict)"() -> ("Value"=w266:bool)  [unwired: 2 in, 2 out]
                          n252 = case shown="True" w266 {
                            frame False {
                              w268 = FALSE ("Ga Active")
                              w267 = 0.0 ("Ga Flow 1")
                              n253 = call "set_Ga.vi"("Ga Active"=w268, "Ga Flow 3"=w267, "Ga Flow 2"=w267, "Ga Flow 1"=w267, "Ga Bubbler"=w268, "Ga H2 Dilute"=w268, "Ga Run"=w268, "Ga Remote"=w268) -> ()  [unwired: 8 out]
                            }
                            frame True {
                              w270 = TRUE ("Ga Active")
                              n254 = property on="Ga Dilution" class="Bool (strict)"() -> ("Value"=w269:bool)  [unwired: 2 in, 2 out]
                              n255 = property on="Run Ga" class="Bool (strict)"() -> ("Value"=w271:bool)  [unwired: 2 in, 2 out]
                              n256 = property on="GAMFC3 set" class="DigNum (strict)"() -> ("Value"=w272:dbl)  [unwired: 2 in, 2 out]
                              n257 = property on="GAMFC2 val" class="DigNum (strict)"() -> ("Value"=w273:dbl)  [unwired: 2 in, 2 out]
                              n258 = case shown="True" w269 {
                                tunnel: [w275 w276] -> w274
                                frame False {
                                n259 = property on="GAMFC1 val" class="DigNum (strict)"() -> ("Value"=w275:dbl)  [unwired: 2 in, 2 out]
                                }
                                frame True {
                                n260 = property on="GAMFC1 set" class="DigNum (strict)"() -> ("Value"=w276:dbl)  [unwired: 2 in, 2 out]
                                }
                              }
                              n261 = call "set_Ga.vi"("Ga Active"=w270, "Ga Flow 3"=w272, "Ga Flow 2"=w273, "Ga Flow 1"=w274, "Ga Bubbler"=w270, "Ga H2 Dilute"=w269, "Ga Run"=w271, "Ga Remote"=w270) -> ()  [unwired: 8 in]
                            }
                          }
                        }
                        frame True {
                        }
                      }
                    }
                    frame #2 {
                      n262 = case shown="False" w277 {
                        frame False {
                          n263 = property on="In?" class="Bool (strict)"() -> ("Value"=w278:bool)  [unwired: 2 in, 2 out]
                          n264 = case shown="True" w278 {
                            frame False {
                              w280 = FALSE ("In Remote")
                              n265 = call "set_In.vi"("Indium Flow"=0.0, "In Remote"=w280, "In Run"=w280, "In Bubbler"=w280, "In Active"=w280) -> ()  [unwired: 5 out]
                            }
                            frame True {
                              w283 = TRUE ("In Run")
                              n266 = property on="Run In" class="Bool (strict)"() -> ("Value"=w281:bool)  [unwired: 2 in, 2 out]
                              n267 = property on="In Flow" class="DigNum (strict)"() -> ("Value"=w282:dbl)  [unwired: 2 in, 2 out]
                              n268 = call "set_In.vi"("Indium Flow"=w282, "In Run"=w281, "In Bubbler"=w283, "In Active"=w283) -> ()  [unwired: 1 in, 5 out]
                            }
                          }
                        }
                        frame True {
                        }
                      }
                    }
                    frame #3 {
                      n269 = case shown="False" w284 {
                        frame False {
                          n270 = property on="PH3?" class="Bool (strict)"() -> ("Value"=w285:bool)  [unwired: 2 in, 2 out]
                          n271 = case shown="False" w285 {
                            frame False {
                              w286 = FALSE ("P_Gas Active")
                              n272 = call "set_P_gas.vi"("P_Gas Active"=w286, "P_Gas Flow"=0.0, "P_Gas In"=w286, "P_Gas H2 In"=w286, "P_Gas Run"=w286, "P_Gas Remote"=w286) -> ()  [unwired: 10 out]
                            }
                            frame True {
                              w290 = TRUE ("P_Gas Active")
                              n273 = property on="P Flow" class="DigNum (strict)"() -> ("Value"=w289:dbl)  [unwired: 2 in, 2 out]
                              n274 = property on="Run P" class="Bool (strict)"() -> ("Value"=w288:bool)  [unwired: 2 in, 2 out]
                              n275 = call "set_P_gas.vi"("P_Gas Active"=w290, "P_Gas Flow"=w289, "P_Gas In"=w290, "P_Gas Run"=w288) -> ()  [unwired: 2 in, 10 out]
                            }
                          }
                        }
                        frame True {
                        }
                      }
                    }
                    frame #4 {
                      n276 = case shown="False" w291 {
                        frame False {
                          n277 = property on="AsH3?" class="Bool (strict)"() -> ("Value"=w292:bool)  [unwired: 2 in, 2 out]
                          n278 = case shown="True" w292 {
                            frame False {
                              w293 = FALSE ("As_Gas Active")
                              n279 = call "set_As_gas.vi"("As_Gas Active"=w293, "As_Gas Flow"=0.0, "As_Gas In"=w293, "As_Gas H2"=w293, "As_Gas Run"=w293, "As_Gas Remote"=w293) -> ()  [unwired: 10 in]
                            }
                            frame True {
                              w296 = TRUE ("As_Gas Active")
                              n280 = property on="Run As" class="Bool (strict)"() -> ("Value"=w295:bool)  [unwired: 2 in, 2 out]
                              n281 = property on="AsH3 Flow" class="DigNum (strict)"() -> ("Value"=w297:dbl)  [unwired: 2 in, 2 out]
                              n282 = call "set_As_gas.vi"("As_Gas Active"=w296, "As_Gas Flow"=w297, "As_Gas In"=w296, "As_Gas Run"=w295) -> ()  [unwired: 12 in]
                            }
                          }
                        }
                        frame True {
                        }
                      }
                    }
                    frame #5 {
                      n283 = call "Set_Argument.vi"("Enable"=TRUE, "Argument"="run_started", "Argument List In"=w299) -> ("Argument List Out"=w298:string[])
                    }
                  }
                }
              }
            }
          }
        }
      }
    }
    frame "End" {
    }
    frame "Idle" {
    }
  }
  "Argument List Out" <- w10
